vi "2022_day2.vi"() -> ()   [LabVIEW 2021]
panel:
  out "Task 2":i32
  out "Task 1":i32
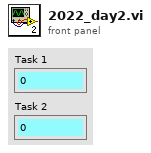
[diagram p1: front panel]
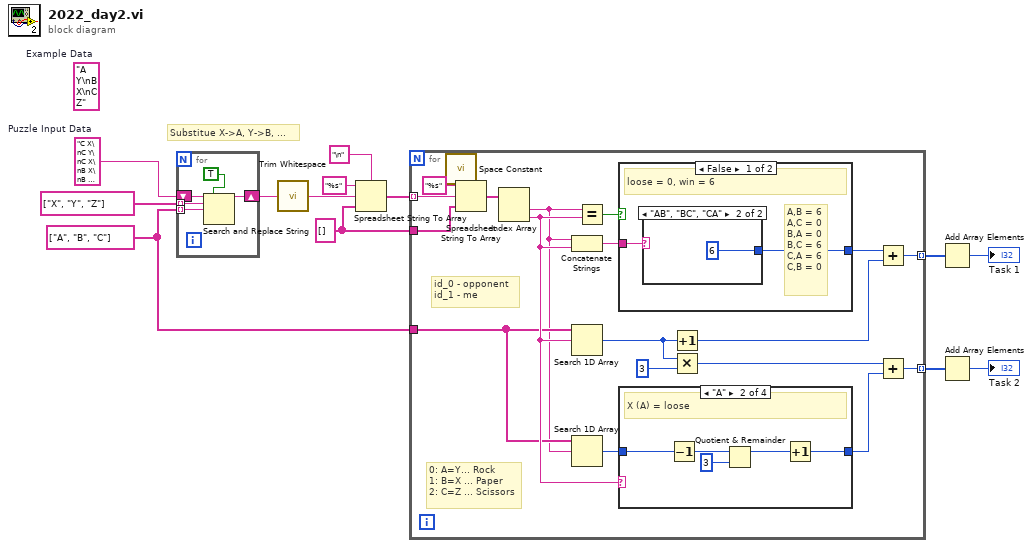
[diagram p0: block diagram]
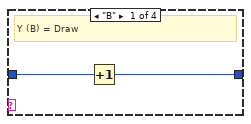
[diagram p2: hidden frame]
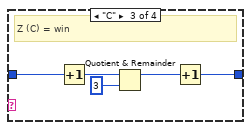
[diagram p3: hidden frame]
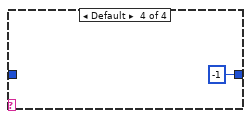
[diagram p4: hidden frame]
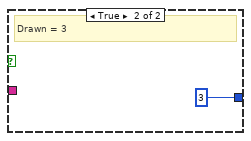
[diagram p6: hidden frame]
diagram:
  w1 = "C X\nC Y\nC X\nB X\nB Z\nA Z\nC Y\nC Z\nB Z\nC X\nB Y\nC Y\nC Y\nA Y\nC Y\nC Y\nC Z\nC X\nB Z\nC Y\nA Y\nA Y\nC Z\nB Y\nA Y\nC Z\nC Y\nA Y\nA Y\nB Y\nC Y\nC Z\nC Y\nB X\nB Z\nC Y\nB Z\nA X\nC Z\nA Y\nB Y\nC Y\nC Y\nB Z\nB Y\nA Z\nC X\nC X\nC Y\nC X\nB Z\nA Y\nB X\nB Z\nC Z\nC X\nC X\nB Z\nA Y\nB Y\nC Y\nC Y\nA Y\nC X\nA Y\nB Z\nC Y\nC Y\nB Y\nC Y\nA Z\nA Z\nB X\nA Y\nC Y\nA Y\nC Y\nC Y\nC X\nC Y\nB Z\nC Y\nC Z\nC X\nB X\nC Y\nC Y\nC X\nC Z\nA Y\nC X\nB Z\nC X\nA Y\nB Y\nC Y\nA Y\nA Y\nA Y\nB Y\nC Y\nA Y\nA Y\nC Z\nC Y\nB Y\nC X\nC Y\nB Z\nB Z\nC X\nC Y\nC X\nC Y\nC Y\nA Y\nC Y\nC X\nC Y\nC Y\nB Y\nB Z\nA Y\nB Y\nA Y\nA Y\nC Y\nB X\nC Y\nC X\nA Y\nC X\nC X\nC Y\nC Y\nB Z\nC X\nA Y\nB Z\nC Z\nC X\nA Y\nB Z\nC Y\nB Y\nA Y\nA Y\nC Y\nB Y\nC Y\nC X\nC Y\nA Y\nC Y\nA Y\nB Y\nC X\nC Y\nC Y\nB Z\nB Z\nA Y\nC Y\nC Y\nC Y\nC Y\nA Y\nC X\nC Z\nC X\nA Y\nA Y\nA Y\nC Y\nB Z\nB Z\nC Y\nC Y\nB X\nC Y\nC Y\nB Z\nB X\nB Y\nC Y\nC Y\nC X\nB Y\nB Z\nB Z\nC Y\nC Y\nC X\nC X\nA Y\nC Y\nC Y\nB X\nB Z\nB X\nB Z\nB Y\nC X\nB X\nB Y\nB Z\nB Z\nB X\nB Z\nB Y\nC X\nC Y\nC X\nC X\nB Z\nC Y\nC Y\nC Y\nB Z\nC Y\nC X\nC Y\nC Y\nA Z\nC Y\nA Y\nC Y\nA Z\nA X\nC Y\nC Y\nC Y\nC Z\nB Z\nB Z\nC Y\nB Z\nB Z\nC X\nC Y\nA Y\nA Y\nC Y\nA Y\nC Y\nC Y\nB Y\nA Y\nC Y\nB Z\nA Y\nB Z\nC X\nC Y\nA Y\nB Z\nA Y\nC X\nC Y\nB Y\nC Y\nA Z\nB Z\nB X\nC Y\nA Y\nA Z\nC X\nA Y\nB Z\nA Y\nB Y\nC Y\nC Y\nB Z\nB Z\nC X\nB Z\nC X\nC Z\nC Y\nC X\nA Y\nC X\nA Y\nA Y\nB Z\nB Z\nB Z\nA Y\nA Y\nC Y\nA Y\nB Z\nC X\nC Y\nC Y\nC Y\nB Y\nA Y\nC Z\nC Y\nA Y\nA Y\nB Z\nC Y\nC Y\nC Y\nB Z\nC Y\nC Y\nA Y\nA Y\nC Y\nC X\nB Z\nB Z\nC X\nC X\nC Z\nA Y\nC Y\nA Y\nA Y\nC X\nA Z\nB Y\nA Y\nC X\nA Y\nC X\nC X\nA Y\nA Y\nC X\nB Y\nB Z\nC Y\nC Z\nC Y\nC Y\nB Z\nC Y\nA Y\nA X\nB Y\nC Y\nA Y\nC Y\nC Y\nC Y\nA Y\nC Y\nA Y\nC Y\nB Z\nA Y\nC X\nC Y\nA Y\nC Y\nA Y\nA Y\nA Y\nB Z\nC Y\nB Z\nA Y\nC Y\nA Y\nC Y\nC X\nB Z\nA Y\nC X\nB Z\nB Y\nC Y\nC Z\nC Y\nB Y\nB Y\nA Y\nA Y\nC X\nB Y\nA Y\nC Y\nB X\nC X\nA Y\nC Y\nA Y\nC Y\nB Z\nA Z\nB Z\nB Z\nA Z\nC Y\nC Y\nC X\nB Y\nC Y\nA Y\nC Y\nC Y\nB Y\nB Z\nC Y\nC X\nA Y\nC X\nC X\nC Y\nB Y\nC Y\nB Z\nC Y\nA Y\nA Y\nC Y\nC X\nC X\nC X\nC Y\nC X\nC Y\nC Y\nA Y\nC Y\nC X\nC Y\nC X\nC X\nC X\nA Y\nB Y\nC Y\nC Y\nC Y\nC Y\nC Y\nA Y\nA X\nB Z\nC X\nC Y\nC Y\nB Z\nA Y\nA Y\nB X\nB Z\nC Y\nC Y\nB Z\nA Y\nA Y\nA Y\nC Y\nC Y\nA Y\nA Y\nC Y\nC Y\nC X\nC X\nC X\nB Z\nC Z\nC X\nA Z\nC Y\nC X\nA Y\nB Y\nB Z\nC X\nC Y\nC Y\nC Z\nC Y\nC X\nA Z\nC Y\nA X\nB Y\nC Y\nC Y\nC Y\nC X\nB Y\nB Y\nC X\nB X\nA Y\nC Y\nC Y\nC Y\nB X\nC Y\nA Y\nC Y\nC Y\nB Z\nC X\nB X\nC Z\nC Y\nA Y\nB Y\nB Z\nC Z\nC X\nC X\nA Y\nA Y\nB Z\nA Y\nC X\nB Y\nC Y\nA Y\nB X\nA Y\nA Y\nC Z\nC Y\nC Z\nB Z\nA X\nC Y\nB Y\nC Y\nB Z\nB Y\nC Y\nA Y\nB Z\nB Z\nC X\nB Z\nC Y\nB Z\nB Z\nC Y\nC Y\nB Z\nC Z\nC Y\nB Z\nC Y\nB X\nA Y\nB Z\nA Y\nC Y\nA Y\nC Y\nC Y\nB Y\nB Z\nB Z\nC Y\nA Y\nB Z\nC X\nC Y\nC Y\nA Y\nC Y\nC Y\nC X\nA Y\nC Y\nC Y\nA Y\nC X\nA Y\nA Y\nA Y\nC Y\nC Y\nA Y\nB Z\nA Y\nB Y\nA Y\nA Y\nC Y\nC Y\nC Z\nA Y\nC Y\nB Z\nA Y\nC Y\nC Z\nC Y\nC Y\nB Z\nC Y\nC Y\nB Z\nB Y\nC Y\nA Y\nC X\nC Y\nC Z\nC Z\nC X\nC X\nC X\nC Z\nC Y\nB Z\nA Y\nB Z\nB Z\nA Y\nC Y\nC Y\nC Y\nB X\nC Y\nA Y\nA Z\nB Y\nB Y\nA Y\nB Z\nA Y\nB Y\nC Z\nC Y\nC Y\nC Y\nB Z\nB Z\nB Z\nC Y\nC Y\nA Y\nC X\nC X\nA Y\nC Y\nC Y\nC Y\nC Y\nC X\nC Y\nC Y\nC Y\nC X\nA Z\nB Y\nC Y\nA Y\nA Y\nB Z\nA Z\nC Y\nC Y\nC Y\nC X\nB X\nB Y\nC Y\nA Y\nA Z\nB X\nC Y\nC Y\nB Z\nA Y\nA Y\nB Z\nB Z\nC Y\nC Y\nC X\nB Y\nB Z\nC Y\nB Y\nC Y\nA Y\nC X\nC X\nB Z\nA Y\nC Y\nB Z\nC X\nC Y\nB Y\nB Z\nA Z\nB Y\nB Y\nC X\nC Y\nA Z\nC X\nC X\nA Y\nA Y\nC X\nA Y\nB Y\nB Z\nA Y\nB Z\nB X\nC Y\nC Y\nC X\nB Z\nA Y\nB Y\nA Y\nC Y\nC Z\nB Z\nC Y\nA Y\nC Y\nC Z\nA Z\nB Z\nB X\nC Y\nC Y\nB Y\nC X\nB Y\nB Z\nB Z\nB X\nB Y\nC X\nC Y\nC X\nC Y\nA Y\nA Y\nC Y\nA Y\nC Y\nC X\nC Y\nA Y\nB Z\nC X\nC Y\nB Z\nC Y\nC Y\nB Y\nB Z\nA X\nC Y\nB Y\nB Y\nB Z\nC Y\nB Z\nA Y\nC Y\nB Y\nC Y\nA Y\nC Y\nB Z\nC Y\nA Y\nA Y\nC Y\nA Y\nC Y\nA Y\nA Y\nB Z\nC X\nC Y\nB Z\nC Y\nA X\nA Z\nC Y\nC X\nC X\nC Y\nC Y\nB Z\nA Z\nA Y\nC Y\nB Z\nA Y\nA Y\nC Y\nB Z\nA Y\nC X\nA Y\nA Y\nC X\nB Z\nB X\nA X\nA Y\nB Y\nA X\nB X\nC X\nC Y\nA Y\nC Y\nA Y\nA Y\nC X\nB Y\nC X\nB Y\nC Y\nC Y\nA Y\nB Z\nA Z\nB Y\nC X\nC Y\nC Y\nB Z\nC Z\nA Y\nA Y\nA Z\nC Y\nA Y\nB Z\nC Y\nC Y\nB Y\nA Y\nA Y\nC Y\nC X\nC X\nB Y\nB Z\nC Y\nB Y\nB Z\nC Y\nA Y\nB Z\nA Y\nA Y\nA Z\nC X\nB Z\nC Y\nB Z\nA Y\nC X\nC Y\nC Y\nB X\nB Z\nA Y\nA Y\nA Y\nA Y\nA Y\nC Y\nA Y\nA Y\nC X\nC Y\nC Z\nB Z\nA Z\nC Z\nA Y\nB Z\nB Y\nA Y\nC Y\nB Z\nA Y\nC Y\nC Y\nA Y\nC Y\nB Z\nB Y\nB Z\nC Y\nC Y\nC Y\nA Z\nC X\nB X\nB Z\nC Z\nC Y\nC Y\nC Y\nC X\nA Y\nC Y\nA Y\nA Y\nB Z\nA Y\nC Y\nC Y\nA Y\nC Y\nA Z\nB X\nA Y\nC Y\nA Y\nA Z\nA Y\nA Y\nB Z\nB Y\nB Z\nC Y\nB Z\nC X\nA Y\nC Y\nA Y\nA Y\nA Y\nB Z\nB Z\nC Y\nB Z\nB Y\nC X\nA Y\nC Y\nA Y\nB Z\nC X\nB Y\nC Y\nB Z\nC Y\nA Y\nC Y\nC Y\nB Y\nB Z\nC Y\nB Z\nB Y\nC Y\nC X\nA Z\nC Z\nC Y\nC Y\nA Y\nA Y\nC X\nC Y\nC Y\nC Y\nC X\nB Z\nC X\nC Y\nA Y\nA Y\nB Z\nA Y\nA Y\nC Y\nA Y\nB Z\nC X\nC Y\nC Y\nC Y\nC Y\nC X\nB Z\nA Y\nB Y\nC Y\nC X\nB Z\nC Y\nA Y\nA Y\nB Z\nC Y\nA Y\nC Z\nC X\nB Z\nC Y\nA Z\nB Z\nA Y\nA Y\nC Y\nB Z\nB Z\nA Y\nC Y\nB Y\nC Y\nA Y\nA Y\nB Y\nB X\nB Z\nC Y\nA Y\nC Y\nA Y\nA Y\nB Z\nB Y\nA Y\nA Y\nA Y\nC Y\nB Y\nC Y\nA Y\nC X\nC Y\nC Y\nB Z\nB Z\nC Y\nC Y\nA Y\nB X\nC X\nA Y\nC Y\nC Y\nC Y\nA Y\nC X\nB Z\nA Y\nC Z\nB Y\nB Y\nC Z\nA Y\nC Z\nC Y\nC X\nB Y\nA Y\nC X\nC X\nC Y\nC X\nC X\nB Z\nC Y\nB Y\nA Y\nB Y\nA Y\nB Z\nC X\nC Y\nC X\nC Z\nC X\nB Z\nC X\nC Y\nC Y\nC Y\nB Z\nA Y\nC Y\nC Y\nC Y\nB Z\nA Y\nC X\nC Y\nC Y\nC Y\nC X\nA Z\nC Y\nC Y\nC X\nB X\nB Z\nA Y\nB Z\nC Y\nB Y\nB Z\nA Y\nB Z\nC Y\nA Y\nA X\nC X\nC X\nC Y\nA Y\nB X\nC Y\nB X\nB Z\nC X\nA Y\nB X\nC X\nA Y\nC Y\nC Y\nC Y\nA Z\nC Y\nA Y\nB Z\nB Z\nA Z\nC Y\nA Y\nB Z\nC Z\nC X\nC X\nC X\nA Y\nA X\nC Y\nA Y\nB Y\nC Y\nC X\nC Y\nC Y\nA Y\nB Z\nC Y\nB Z\nA Y\nC X\nC Y\nB Z\nC Y\nC Y\nB Y\nA Y\nA Y\nA Z\nC Y\nB Z\nB Y\nB Z\nB Y\nA Y\nC Y\nC Y\nC X\nC Y\nC Y\nB Z\nC Y\nC Y\nC X\nB Y\nB Z\nC Y\nC Y\nA Y\nC Z\nC Y\nB Z\nA Y\nA X\nA Y\nC X\nC Y\nC Y\nB Z\nA Y\nB X\nC Z\nC Z\nC X\nC Y\nB Z\nC Z\nB Z\nC Y\nA Y\nC Y\nA Y\nB X\nC X\nC Y\nB Z\nC Y\nB Y\nB X\nB X\nB Z\nC Y\nC Y\nB Y\nB Z\nC Y\nA Y\nB Z\nC Y\nB Z\nC Y\nB Z\nC Y\nA Y\nA Y\nC Y\nC Y\nB Y\nB Z\nC Y\nB Z\nC X\nB Z\nC Y\nB X\nC X\nB Z\nA Y\nC X\nB Z\nC Y\nA Y\nB Z\nA X\nB Z\nB Z\nB Z\nC Y\nC Y\nC Y\nC Y\nA Y\nA Y\nB Z\nB X\nC X\nC Y\nB Y\nA Y\nA Y\nB Z\nC Y\nA Y\nA Y\nC Y\nC X\nC Y\nC X\nC Y\nC Y\nC Y\nB Z\nC Y\nC X\nB Y\nC Y\nC Y\nC Y\nA Z\nC X\nC Y\nA Y\nC Y\nB Z\nB Y\nC Y\nA Y\nA Y\nC Y\nC Y\nC X\nA Y\nC Y\nA Z\nA Y\nB Z\nA Y\nC X\nC Y\nC Y\nB X\nB Z\nC X\nB X\nC Z\nC X\nB Z\nB Z\nC Y\nC X\nB Z\nB Z\nB Z\nC Y\nC Y\nA Y\nC Y\nB Y\nB X\nC Y\nC Y\nC Y\nB X\nC X\nB X\nC Y\nA Y\nC Y\nC X\nC Y\nC Y\nB X\nB Z\nA Z\nB Z\nA Y\nB Z\nC X\nB Z\nC Y\nC Y\nC Z\nA Y\nC Y\nC Y\nA Z\nB Y\nC Y\nA X\nA Y\nB Y\nC Y\nB Z\nC Y\nC X\nC Y\nB Z\nA Y\nC X\nC Y\nC X\nC Y\nC Y\nC Z\nA Y\nC Y\nB Z\nA Y\nC Z\nC Y\nA Y\nC Y\nC Y\nC Y\nC Y\nA Y\nC Y\nC Y\nC Y\nC Y\nB Z\nC X\nA Y\nA Y\nC Y\nB Y\nC Y\nC Y\nA Z\nC Y\nB Y\nC Y\nB Z\nC X\nA Y\nC Y\nC Y\nB Z\nC Y\nA Y\nA Y\nC Y\nB Z\nC Y\nA Y\nB Z\nC Y\nC Y\nB Z\nC X\nB Z\nB Z\nC Y\nC Y\nA Y\nC X\nA Y\nC Y\nB Z\nA Y\nB Z\nA Y\nC X\nC Y\nB Z\nB Y\nB Z\nA Y\nB Z\nC Y\nB Z\nC Y\nB Y\nA Y\nB Z\nB X\nB Z\nC Y\nB Z\nB Z\nB Z\nA Y\nA Y\nC Y\nB Z\nB Z\nC X\nB Z\nC Z\nA Y\nB Z\nB Z\nC Y\nB Z\nB Z\nC X\nC Z\nA Z\nC Y\nC Y\nB X\nC Z\nC Y\nA Y\nB Z\nC X\nB Z\nC Y\nC Y\nB Z\nB Z\nB Z\nC X\nC Y\nC X\nC X\nA Y\nB Z\nB Y\nC Y\nC Y\nB Z\nC Y\nC Y\nC Y\nC Y\nC Y\nB X\nA Y\nA Y\nB Y\nC Y\nB Y\nC Y\nB Y\nB Z\nC Y\nC Y\nC X\nB Y\nA Y\nB X\nB Z\nC X\nA X\nC Y\nA Y\nA Y\nC X\nB Y\nA Y\nB Z\nC X\nB Z\nC Z\nC X\nC Y\nC X\nC Y\nC Y\nC Y\nB Y\nC Z\nC X\nB Z\nC Y\nC X\nC X\nB Y\nC Y\nC Y\nC Z\nB Z\nC Y\nC Y\nB Y\nC Z\nC X\nB Z\nC Y\nC X\nC Y\nB Z\nC Y\nC Y\nA Y\nB Y\nC X\nC Y\nC Y\nC Y\nB Y\nB Y\nC Z\nB Z\nC Y\nB Z\nA Z\nC X\nB X\nC X\nA Y\nC Y\nA Z\nC X\nC Y\nA Y\nA Y\nB Y\nA Y\nC Y\nB Y\nC X\nC X\nC X\nC X\nC Y\nC Y\nA Y\nB Z\nC Y\nA Z\nC Y\nA Y\nB Z\nB Z\nC Y\nA Z\nC Y\nC Y\nC Y\nB Z\nC Y\nC Y\nA X\nA Y\nA Z\nC Y\nA Y\nB X\nA Y\nB Z\nB Y\nB Z\nB Y\nC X\nC X\nA Y\nB Z\nB Y\nC X\nB X\nB Y\nA Y\nC Y\nC Y\nC Y\nB Z\nC Y\nA Y\nB Z\nC X\nB Z\nB Z\nB X\nB Y\nC Y\nC Y\nC X\nB Z\nC Y\nC Y\nC Y\nA Y\nC Y\nB Z\nB Y\nC Y\nC X\nC X\nB X\nB Z\nA Z\nC X\nA Y\nB Y\nC Y\nA Y\nB Y\nC Y\nC Y\nC Z\nC Y\nC X\nA Y\nC Y\nC Y\nB Z\nC Y\nC Y\nC Y\nC Y\nA Y\nB Z\nB Z\nC Y\nC Y\nC Y\nC Y\nC Y\nB Z\nC Y\nC Y\nC X\nA Y\nA Y\nC Y\nC X\nA Y\nB Z\nA Y\nC X\nC Y\nC Z\nC Y\nA Z\nA Y\nA Y\nB Y\nC Y\nC Y\nB Y\nC Y\nA Y\nC X\nB Z\nC X\nA Y\nB Z\nC X\nA Y\nC X\nC X\nA Z\nA Y\nB Y\nA Y\nB Y\nA Z\nC Y\nC Y\nC Y\nB Z\nC Y\nA Y\nB Z\nB Y\nC Y\nB Y\nC Z\nA Y\nB Y\nC Y\nB Y\nA Y\nB Z\nC Y\nC X\nC Y\nA Y\nA Z\nC Y\nB Z\nC Y\nB Y\nA Y\nC X\nA Z\nC Z\nC X\nA Y\nC X\nC X\nC Y\nC Z\nA Y\nA Y\nC Y\nA Y\nC Y\nB Z\nC X\nA X\nC X\nC Y\nC Y\nC Y\nC Y\nB Z\nB Z\nB Z\nC X\nC Y\nB Y\nC Y\nB Y\nC Z\nA X\nB Y\nC X\nB Y\nC X\nB Y\nC Y\nB Z\nC X\nA Y\nB Z\nC X\nA X\nC Y\nB Z\nB Z\nC X\nB Z\nB Z\nC X\nC Y\nC Z\nB Z\nC Y\nC Y\nC Y\nB X\nA Y\nB Y\nB Z\nB Z\nC X\nA Z\nC Y\nC Y\nA Y\nA X\nA Y\nC Y\nB Y\nC Y\nA Y\nC X\nC Y\nC Y\nC Y\nC Y\nC Y\nC Y\nC Y\nC Y\nC Y\nC Y\nB Z\nB Z\nA Y\nB Y\nC Y\nC Y\nC X\nB Z\nA Y\nC Y\nB Z\nC Y\nA Y\nC X\nB X\nC Z\nA Y\nC X\nB Y\nC X\nB Z\nA Y\nC Y\nC Y\nC Y\nB Z\nB Z\nA Z\nC Z\nA Y\nB Z\nC X\nC Y\nA Y\nC Y\nC Y\nC X\nB Z\nC Z\nC Y\nB Z\nA X\nB Y\nA Z\nB X\nC X\nA Y\nC Y\nB Z\nB Z\nC Y\nA Y\nB Z\nB Z\nA Y\nA Y\nB Z\nB Z\nA X\nB Z\nC Y\nC Z\nC Y\nC Y\nB Z\nC Y\nA Z\nA X\nC X\nB Y\nB Z\nC X\nB Z\nA X\nA Y\nA Y\nB X\nB Y\nB Z\nC X\nC X\nC X\nC Y\nC Y\nB X\nC Y\nC Y\nA Y\nC X\nA Y\nB Z\nA Y\nC Y\nB X\nC X\nC Y\nA Y\nC X\nC Y\nC Y\nB Z\nA Y\nA Y\nA Z\nC Y\nB Z\nA Z\nB X\nA Z\nC Y\nB X\nA Y\nC Y\nC Z\nA Z\nC X\nA Y\nB X\nC Y\nC Y\nC X\nC Z\nA Y\nA Y\nC Y\nB Z\nC Y\nC X\nB X\nA Y\nB Y\nB Z\nB Z\nC Y\nC Y\nA Y\nB Z\nB Z\nC Y\nC Z\nC Y\nC Y\nC X\nC X\nA Y\nB Z\nA Y\nB Z\nB Z\nC X\nB X\nC X\nC Y\nB X\nB Z\nC X\nC X\nC X\nB Z\nB Y\nB Z\nC Y\nC Y\nB Z\nB Y\nB Z\nC Y\nB Y\nA Y\nA Y\nB Y\nA Y\nB Z\nA Y\nC X\nA Y\nC Z\nB Y\nC Y\nC X\nC X\nC Y\nC X\nC Y\nA Y\nB Z\nC X\nC Y\nC Y\nC Y\nC Y\nC Y\nB Y\nA Y\nB Z\nC Y\nA Z\nC Y\nB Z\nC X\nC Z\nA Y\nB Z\nC X\nC Y\nB Z\nC Y\nA Y\nC Y\nC X\nC X\nC Y\nA Y\nB Y\nA X\nC Y\nC Y\nA Y\nC Y\nA X\nC Y\nB Y\nC X\nB Z\nB Z\nB Y\nC Y\nC Z\nC X\nB Z\nB Z\nB Y\nC Z\nA Y\nC Y\nC Y\nB Y\nC X\nA Y\nC Y\nC Y\nA Z\nA Y\nB Y\nC Y\nC Y\nC X\nB X\nC Y\nA Y\nB Z\nB Y\nA Y\nB Y\nC Y\nC X\nC Y\nC Y\nC X\nA Y\nB Z\nC X\nC Z\nB X\nC Y\nC X\nC Y\nC X\nC Y\nB Z\nA Y\nA Y\nB Z\nC Y\nC Y\nB Z\nC Y\nC X\nB Z\nC Y\nB Z\nC X\nC Y\nC X\nA Y\nC Y\nA X\nC Y\nC X\nA Y\nC Y\nA Y\nC Y\nA Y\nC X\nA Y\nA Y\nA Y\nB Y\nB Z\nC Y\nB Z\nA Y\nC Y\nC X\nB X\nC Y\nB Z\nB X\nB X\nB Y\nC Y\nC X\nC Y\nC X\nB Y\nB Z\nA Y\nB Y\nC Y\nC Z\nA Y\nC Y\nB Y\nA Y\nC X\nC Y\nA Y\nC Y\nA Z\nC Z\nC Y\nB Z\nC Y\nC Y\nB Y\nA Y\nC Z\nA X\nC Y\nB Z\nC Z\nB X\nC Y\nC X\nC X\nB Z\nB Z\nB X\nB Y\nC Y\nB Z\nB Z\nB Z\nA Y\nB Z\nC Y\nC Y\nA Y\nA X\nC Z\nA Y\nC Z\nC Y\nC X\nC Y\nC X\nB Z\nC Y\nA X\nB Z\nB Y\nC Y\nB Y\nC Y\nC Y\nA Y\nB Z\nB Y\nC Y\nC X\nC Y\nC Y\nB Z\nA Y\nB X\nC Y\nC Y\nC Y\nA Y\nC Y\nC Y\nC X\nC Z\nC X\nB Y\nA Y\nC Z\nB Z\nB Z\nA Y\nC Y\nC X\nB X\nC X\nB Z\nA Y\nC Y\nC Y\nB Z\nA Y\nB Y\nC X\nB Y\nB Z\nB Z\nB Z\nB X\nB Y\nB Z\nC X\nA Z\nA Y\nC Y\nA Y\nC Y\nC Y\nB Z\nB Z\nC X\nB X\nC Y\nA Z\nC Y\nC X\nC Y\nB Y\nC X\nB Z\nC Y\nC X\nB Z\nA Y\nA Y\nC Y\nA Y\nA Z\nC Y\nA Z\nA Y\nC Y\nC X\nB X\nC Y\nC Y\nC X\nA Y\nC X\nC Y\nB Z\nB X\nC Y\nA Y\nB X\nC Y\nB Y\nC X\nA Y\nB Z\nC Y\nC Y\nB Z\nA Y\nA Z\nC Y\nC Y\nC X\nA Y\nB Z\nB Z\nB Y\nB Z\nA Y\nC Y\nA Y\nB Y\nA Y\nC X\nC Y\nA Z\nA Z\nB Y\nA Y\nC Y\nA X\nC Y\nC Y\nB Z\nC Y\nC X\nC Y\nA Y\nC Y\nC Y\nC Y\nC Y\nA X\nC Y\nB Y\nC Y\nA Y\nC Y\nC X\nC X\nC Z\nB Z\nA Y\nB X\nC Y\nC Y\nC Y\nA Y\nB Z\nB Z\nC Y\nA Y\nB Z\nA Y\nC X\nC X\nA Y\nC Z\nC Y\nB Z\nB Z\nA Y\nA Y\nC Y\nA Y\nC Y\nA Y\nB Z\nC X\nC Y\nC Y\nA Y\nC Y\nA Y\nA Z\nB Y\nC Y\nC X\nA Y\nC X\nA X\nC Y\nC Y\nB Y\nC Y\nB Z\nA Y\nC X\nB Z\nA Y\nC X\nB Z\nA Y\nC Y\nB Z\nA Y\nB Z\nC X\nC Y\nC X\nC Y\nB Z\nC Y\nB Y\nC Z\nB Z\nC Y\nC Y\nA X\nC X\nA Y\nC Y\nB Z\nA Y\nA Z\nB Z\nC Y\nC Y\nA Y\nA Y\nA Y\nC X\nC Y\nA Z\nC Y\nC Z\nA Y\nA Y\nC Y\nC X\nC X\nC Z\nC Y\nC Z\nB Z\nA Y\nB Z\nB Z\nC X\nA Y\nB Y\nA Y\nA Z\nA Y\nC Y\nC Y\nC Z\nA Y\nC Y\nB Y\nC X\nC X\nB X\nC Y\nA Y\nC Z\nA Y\nB Z\nB Y\nC Y\nA Y\nA Y\nC Y\nC Y\nC Y\nC Y\nC Y\nC Y\nC Y\nA Y\nB Y\nA Y\nB Y\nB Y\nC X\nC X\nC Y\nA Y\nC Y\nC Y\nC Z\nC Y\nC Y\nB Y\nC Y\nB Y\nA Y\nC Y\nB Z\nC X\nC Y\nA Z\nA Z\n"  # Puzzle Input Data
  (unwired) "A Y\nB X\nC Z"  # Example Data
  w5 = string[] ["A", "B", "C"] ("array type (2D Dbl)")
  w4 = string[] [] ("array type (2D Dbl)")
  # "Substitue X->A, Y->B, ..."
  n1 = for {
    shift-right: [w16] -> w8
    shift-left: w1 -> [w18]
    tunnel: string[] ["X", "Y", "Z"] ("array type (2D Dbl)") -> [w15] mode=indexing
    tunnel: w5 -> [w14] mode=indexing
    n2 = Search and Replace String(replace all?=TRUE ("replace all? (F)"), input string=w18, search string=w15, replace string=w14) -> (result string=w16:string)  [unwired: 4 in, 3 out]
  }
  n3 = call <vilib>:"Trim Whitespace.vi"("string"=w8) -> ("trimmed string"=w11:string)  [unwired: 1 in]
  n4 = Spreadsheet String To Array(delimiter (Tab)="\n", format string="%s", spreadsheet string=w11, array type (2D Dbl)=w4) -> (array=w10:string[])
  n5 = for {
    tunnel: w10 -> [w37] mode=indexing
    tunnel: w4 -> [w34]
    tunnel: [w30] -> w7 mode=indexing
    tunnel: w5 -> [w22]
    tunnel: [w25] -> w2 mode=indexing
    # "0: A=Y... Rock\n1: B=X ... Paper\n2: C=Z ... Scissors"
    # "id_0 - opponent\nid_1 - me"
    n6 = call <vilib>:"Space Constant.vi"() -> ("String"=w36:string)
    n7 = Spreadsheet String To Array(delimiter (Tab)=w36, format string="%s", spreadsheet string=w37, array type (2D Dbl)=w34) -> (array=w33:string[])
    n8 = Index Array(array=w33) -> (element #1=w21:string, element #2=w27:string)  [unwired: 2 in]
    n9 = Concatenate Strings(w21, w27) -> (w28:string)
    n10 = Search 1D Array(1D array=w22, element=w27) -> (index of element=w24:i32)  [unwired: 1 in]
    n11 = Search 1D Array(1D array=w22, element=w21) -> (index of element=w20:i32)  [unwired: 1 in]
    n12 = Equal?(x=w21, y=w27) -> (x = y?=w32:bool)
    n13 = case shown="False" w32 {
      tunnel: w28 -> [w52 _]
      tunnel: [w51 3] -> w31
      frame False {
        # "A,B = 6\nA,C = 0\nB,A = 0\nB,C = 6\nC,A = 6\nC,B = 0"
        # "loose = 0, win = 6"
        n14 = case shown="\"AB\", \"BC\", \"CA\"" w52 {
          tunnel: [_ 6] -> w51
          frame Default {
          }
          frame "AB", "BC", "CA" {
          }
        }
      }
      frame True {
        # "Drawn = 3"
      }
    }
    n15 = case shown="\"A\"" w27 {
      tunnel: [w39 w44 w49 -1] -> w23
      tunnel: w20 -> [w38 w43 w48 _]
      frame "B" {
        # "Y (B) = Draw"
        n16 = Increment(x=w38) -> (x+1=w39:i32)
      }
      frame "A" {
        # "X (A) = loose"
        n17 = Decrement(x=w43) -> (x-1=w41:i32)
        n18 = Quotient & Remainder(x=w41, y=3) -> (x-y*floor(x/y)=w40:i32)  [unwired: 1 out]
        n19 = Increment(x=w40) -> (x+1=w44:i32)
      }
      frame "C" {
        # "Z (C) = win"
        n20 = Increment(x=w48) -> (x+1=w46:i32)
        n21 = Quotient & Remainder(x=w46, y=3) -> (x-y*floor(x/y)=w45:i32)  [unwired: 1 out]
        n22 = Increment(x=w45) -> (x+1=w49:i32)
      }
      frame Default {
      }
    }
    n23 = Increment(x=w24) -> (x+1=w29:i32)
    n24 = Multiply(x=w24, y=3) -> (x*y=w19:i32)
    n25 = Add(x=w31, y=w29) -> (x+y=w30:i32)
    n26 = Add(x=w19, y=w23) -> (x+y=w25:i32)
  }
  n27 = Add Array Elements(numeric array=w7) -> (sum=→"Task 1":i32)
  n28 = Add Array Elements(numeric array=w2) -> (sum=→"Task 2":i32)
